vi "FTW-HTTPClient-OpenConnection.vi"(0 "Username":string, 5 "Password":string, 7 "Timeout (10000msec)":i32=10000, 9 "Trusted Server CA Certificate":path, 11 "error in":errorcluster, 12 "Verify Server Certificate?":bool=TRUE) -> (4 "HTTP Client":refnum<class "FTW-HTTPClient.lvclass">, 15 "error out":errorcluster)   [LabVIEW 2012, in "FTW-HTTPClient.lvclass"]
uses:
  FTW-HTTPClient.lvclass
  FTW-HTTPClient.lvclass/FTW-HTTPClient.ctl
panel:
  # "Inputs"
  # "Outputs"
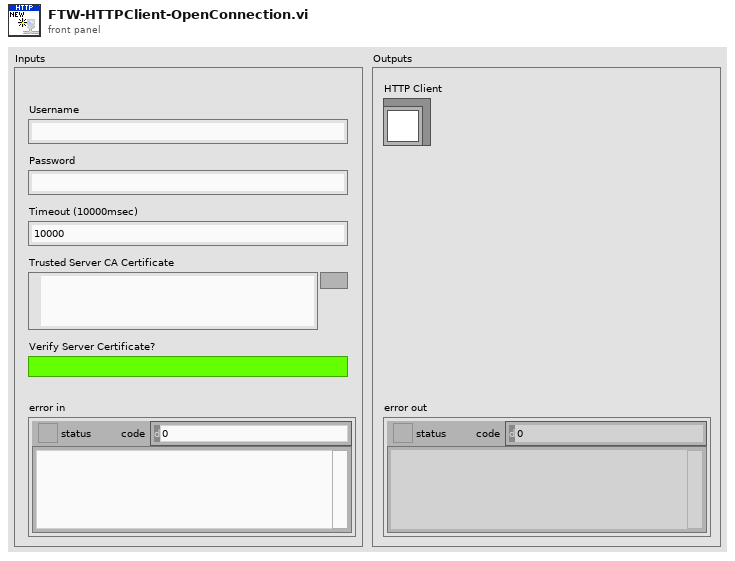
[diagram p1: front panel]
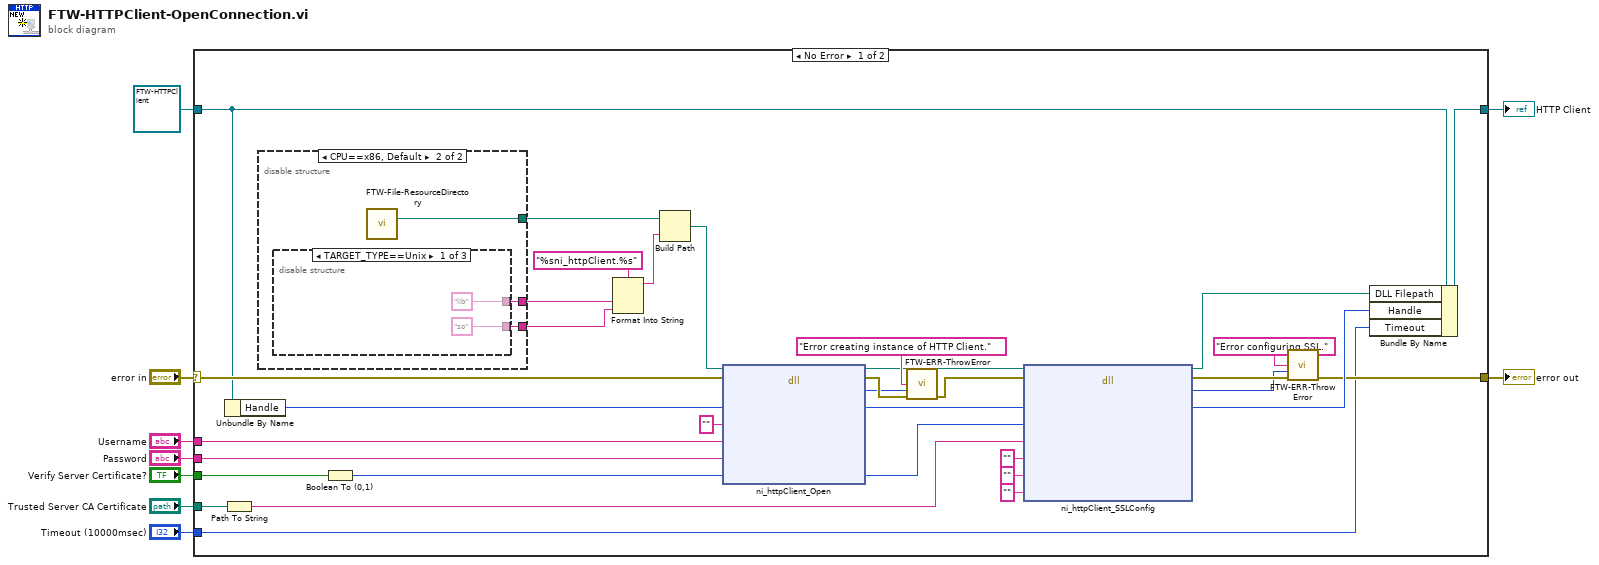
[diagram p0: block diagram]
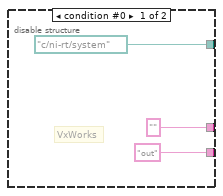
[diagram p2: hidden frame]
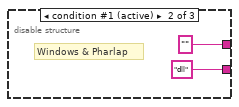
[diagram p3: hidden frame]
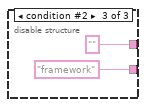
[diagram p4: hidden frame]
diagram:
  n1 = case shown="No Error" "error in" {
    selector: "error in" -> [w37 w57]
    tunnel: "Username" -> [w35 _]
    tunnel: "Password" -> [w34 _]
    tunnel: [w22 w57] -> w7
    tunnel: refnum<class "FTW-HTTPClient.lvclass"> refnum ("HTTP Client") -> [w33 w56]
    tunnel: "Trusted Server CA Certificate" -> [w19 _]
    tunnel: [w43 w56] -> w4
    tunnel: "Timeout (10000msec)" -> [w10 _]
    tunnel: "Verify Server Certificate?" -> [w14 _]
    frame No Error {
      n2 = Path To String(path=w19) -> (string=w18:string)
      n3 = Unbundle By Name(w33) -> ("Handle"=w32:u32)
      n4 = disable-structure shown="CPU==x86, Default" {
        disable-tunnel: ["out" w49] -> w39
        disable-tunnel: ["" w48] -> w40
        disable-tunnel: [path "c:/ni-rt/system" w47] -> w42
        frame condition #0 {
          # "VxWorks"
        }
        frame condition #1 (active) {
          n5 = disable-structure shown="TARGET_TYPE==Unix" {
            disable-tunnel: ["so" ("name or relative path") "dll" "framework"] -> w49
            disable-tunnel: ["lib" "" ""] -> w48
            frame condition #0 {
            }
            frame condition #1 (active) {
              # "Windows & Pharlap"
            }
            frame condition #2 {
            }
          }
          n6 = call "FTW-File-ResourceDirectory.vi"() -> ("Resource"=w47:path)  [unwired: 11 in, 4 out]
        }
      }
      n7 = Boolean To (0,1)(Boolean=w14) -> (0, 1=w12:i16)
      n8 = Format Into String(format string="%sni_httpClient.%s" ("name or relative path"), w40, w39) -> (resulting string=w38:string)  [unwired: 2 in, 1 out]
      n9 = Build Path(base path=w42, name or relative path=w38) -> (appended path=w31:path)
      n10 = dll-call lib="?" fn="ni_httpClient_Open"(path in=w31, error in=w37, "Handle"=w32, "Cookie Filepath"="", "Username"=w35, "Password"=w34, "Verify Server"=w12) -> (path out=w11:path, error out=w30:errorcluster, "Return"=w29:i32, "Handle"=w25:u32, "Verify Server"=w13:i32)  [unwired: 4 in]
      n11 = call "FTW-ERR-ThrowError.vi"("Error Message"="Error creating instance of HTTP Client.", "Error Code"=w29, "error in"=w30) -> ("error out"=w27:errorcluster)  [unwired: 12 in]
      n12 = dll-call lib="?" fn="ni_httpClient_SSLConfig"(path in=w11, error in=w27, "Handle"=w25, "Verify Server"=w13, "CA Cert Filepath"=w18, "Private Key Filepath"="", "Private Key Password"="", "Client Cert Filepath"="") -> (path out=w26:path, error out=w23:errorcluster, "Return"=w21:i32, "Handle"=w24:u32)  [unwired: 6 in]
      n13 = call "FTW-ERR-ThrowError.vi"("Error Message"="Error configuring SSL.", "Error Code"=w21, "error in"=w23) -> ("error out"=w22:errorcluster)  [unwired: 12 in]
      n14 = Bundle By Name(cluster=w33, "DLL Filepath"=w26, "Handle"=w24, "Timeout"=w10) -> (w43:refnum<class "FTW-HTTPClient.lvclass">)
    }
    frame Error {
    }
  }
  "error out" <- w7
  "HTTP Client" <- w4
